vi "左移动.vi"(3 "移动前":u16[][](array[numeric])) -> (0 "移动后":i32[][](array[numeric]), 1 "分数":ext)   [LabVIEW 8.6]
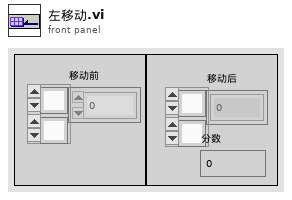
[diagram p1: front panel]
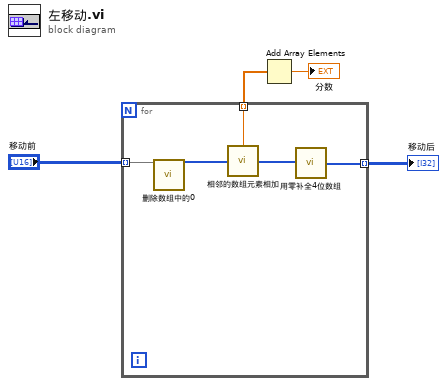
[diagram p0: block diagram]
diagram:
  n1 = for {
    tunnel: "移动前" -> [w9] mode=indexing
    tunnel: [w8] -> w3 mode=indexing
    tunnel: [w5] -> w2 mode=indexing
    n2 = call "删除数组中的0.vi"("数组输入"=w9) -> ("数组输出"=w7:u16[])  [unwired: 10 in]
    n3 = call "相邻的数组元素相加.vi"("数组输入"=w7) -> ("数组输出"=w6:i32[], "分数"=w5:ext)  [unwired: 2 in]
    n4 = call "用零补全4位数组.vi"("数组输入"=w6) -> ("数组输出"=w8:i32[])
  }
  "移动后" <- w3
  n5 = Add Array Elements(numeric array=w2) -> (sum=→"分数":ext)
